vi "MAG_OFFSET.vi"(0 "VISA IN":refnum<visa-resource-name>, 1 "Measurement":string="CH1_S11_1", 3 "Offset Value(dB)":i32, 4 "Offset Slope(dB/1GHz)":i32, 5 "error in":errorcluster, 7 "Channel":i32=1) -> (14 "VISA Out":refnum<visa-resource-name>, 19 "error out":errorcluster)   [LabVIEW 2018, in "PNA-X.lvlib"]
uses:
  PNA-X.lvlib
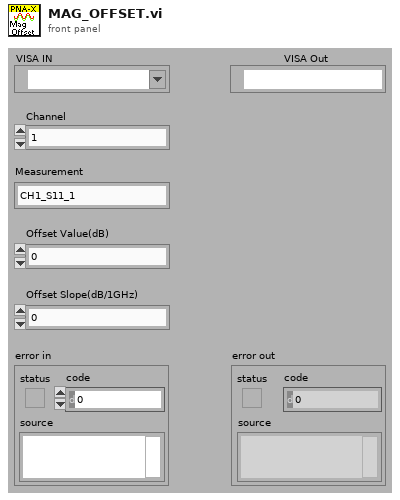
[diagram p1: front panel]
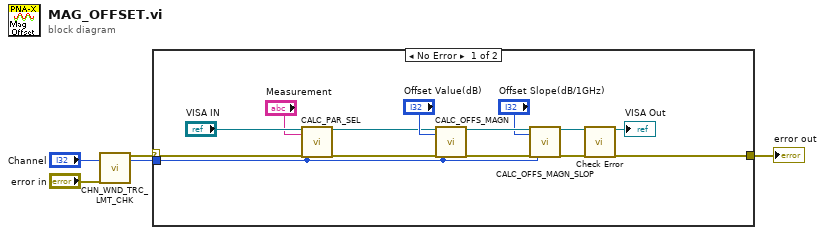
[diagram p0: block diagram]
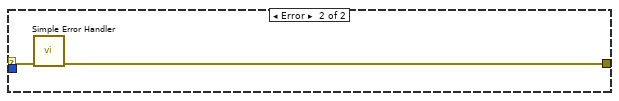
[diagram p2: hidden frame]
diagram:
  n1 = call "CHN_WND_TRC_LMT_CHK.vi"("Channel"="Channel", "error in"="error in") -> ("error out"=w2:errorcluster, "Channel"=w1:i32)  [unwired: 13 in, 3 out]
  n2 = case shown="No Error" w2 {
    selector: w2 -> [w11 w21]
    tunnel: [w19 w20] -> w4
    tunnel: w1 -> [w9 _]
    frame No Error {
      n3 = call "CALC_PAR_SEL.vi"("VISA IN"="VISA IN", "Measurement"="Measurement", "error in"=w11, "Channel"=w9) -> ("VISA Out"=w7:refnum<visa-resource-name>, "error out"=w10:errorcluster)  [unwired: 14 in]
      n4 = call "CALC_OFFS_MAGN.vi"("VISA IN"=w7, "Offset Value(dB)"="Offset Value(dB)", "error in"=w10, "Channel"=w9) -> ("VISA Out"=w15:refnum<visa-resource-name>, "error out"=w17:errorcluster)  [unwired: 14 in]
      n5 = call "CALC_OFFS_MAGN_SLOP.vi"("VISA IN"=w15, "Offset Slope(dB/1GHz)"="Offset Slope(dB/1GHz)", "error in"=w17, "Channel"=w9) -> ("VISA Out"=w14:refnum<visa-resource-name>, "error out"=w16:errorcluster)  [unwired: 14 in]
      n6 = call "Check Error.vi"("VISA Resource Name"=w14, "error in (no error)"=w16) -> ("dup VISA session"=→"VISA Out":refnum<visa-resource-name>, "error out"=w19:errorcluster)  [unwired: 16 in]
    }
    frame Error {
      n7 = call <vilib>:"Simple Error Handler.vi"("error in (no error)"=w21) -> ("error out"=w20:errorcluster)  [unwired: 4 in, 4 out]
    }
  }
  "error out" <- w4
